vi "ADC-NEW.vi"(0 "Analog_Data(V)":dbl=0.0001 min=-15.0 max=30.0 step=0.01, 5 "Voltage_Range(V)":dbl=1.0 min=1e-06 max=30.0 step=0.01, 7 "Resolution (bits)":i32=1 min=1 max=128, 11 "Stop":bool) -> (4 "Digital_Code":i64)   [LabVIEW 2023]
doc: "This VI converts analog value into Digital value."
panel:
  # "ADC"
  # "NOTE:\n This ADC system converts -V to +V and represent the respective Digital code from -(2^(n-1)-1) to (2^(n-1)).\n\nWhere n represent the Resolution (converted for which type of system, eg 8bit, 16bit, 32bit or 64bit systems)"
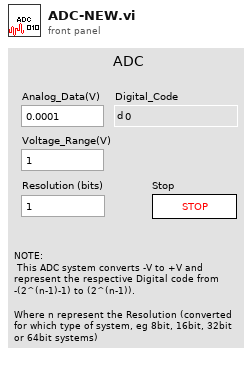
[diagram p1: front panel]
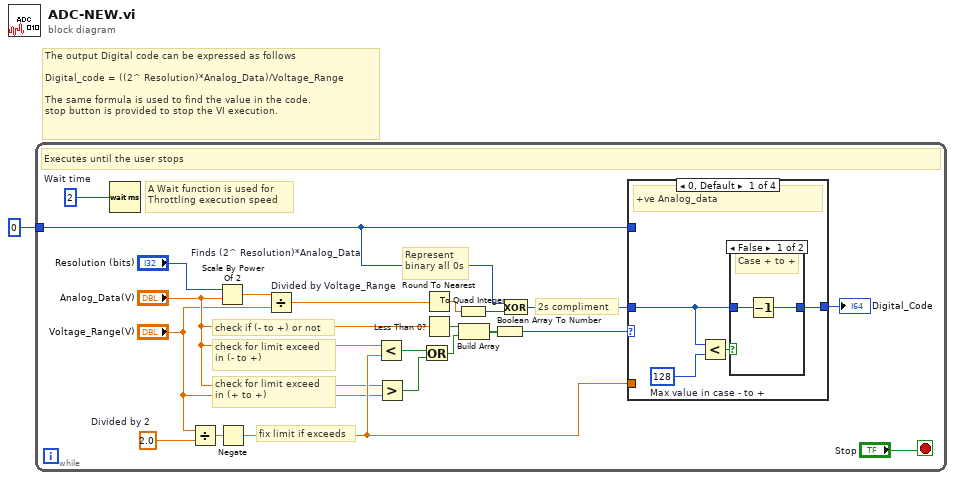
[diagram p0: block diagram]
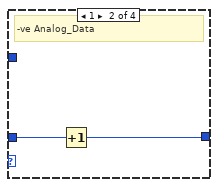
[diagram p3: hidden frame]
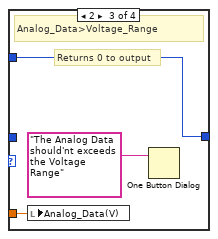
[diagram p4: hidden frame]
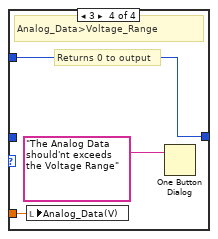
[diagram p5: hidden frame]
diagram:
  # "The output Digital code can be expressed as follows\n\nDigital_code = ((2^ Resolution)*Analog_Data)/Voltage_Range\n\nThe same formula is used to find the value in the code.\nstop button is provided to stop the VI execution."
  n1 = while {
    tunnel: i64 0 -> [w2]
    stop <- "Stop" stop-if-true
    w15 = 2.0  # Divided by 2
    w22 = u32 2  # Wait time
    # "Represent binary all 0s"
    # "check for limit exceed \nin (+ to +)"
    # "check for limit exceed \nin (- to +)"
    # "fix limit if exceeds"
    # "check if (- to +) or not"
    # "2s compliment"
    # "A Wait function is used for \nThrottling execution speed"
    # "Executes until the user stops"
    n2 = Wait (ms)(milliseconds to wait=w22) -> ()  [unwired: 1 out]
    n3 = Divide(x="Voltage_Range(V)", y=w15) -> (x/y=w10:dbl)
    n4 = Scale By Power Of 2 "Finds (2^ Resolution)*Analog_Data"(n="Resolution (bits)", x="Analog_Data(V)") -> (x*2^n=w18:dbl)
    n5 = Negate(x=w10) -> (-x=w7:dbl)
    n6 = Divide "Divided by Voltage_Range"(x=w18, y="Voltage_Range(V)") -> (x/y=w19:dbl)
    n7 = Less?(x="Analog_Data(V)", y=w7) -> (x < y?=w8:bool)
    n8 = Greater?(x="Analog_Data(V)", y="Voltage_Range(V)") -> (0:w3:bool)
    n9 = Or(x=w8, y=w3) -> (x .or. y?=w4:bool)
    n10 = Round To Nearest(number=w19) -> (nearest integer value=w20:dbl)
    n11 = Less Than 0?(x="Analog_Data(V)") -> (x < 0?=w14:bool)
    n12 = To Quad Integer(1:w20) -> (0:w9:i64)
    n13 = Build Array(w14, w4) -> (w13:bool[])
    n14 = Boolean Array To Number(Boolean array=w13) -> (number=w12:u32)
    n15 = Exclusive Or(1:w9, 2:w2) -> (0:w16:i64)
    n16 = case shown="0, Default" w12 {
      tunnel: w16 -> [w24 w31 _ _]
      tunnel: w7 -> [_ _ w33 w36]
      tunnel: [w26 w30 w32 w35] -> w11
      tunnel: w2 -> [_ _ w32 w35]
      frame 0, Default {
        w23 = i64 128  # Max value in case - to +
        # "+ve Analog_data"
        n17 = Less?(x=w24, y=w23) -> (x < y?=w25:bool)
        n18 = case shown="False" w25 {
          tunnel: [w27 w29] -> w26
          tunnel: w24 -> [w28 w29]
          frame False {
            # "Case + to +"
            n19 = Decrement(x=w28) -> (x-1=w27:i64)
          }
          frame True {
            # "Case - to+"
          }
        }
      }
      frame 1 {
        # "-ve Analog_Data"
        n20 = Increment(x=w31) -> (x+1=w30:i64)
      }
      frame 2 {
        # "Returns 0 to output"
        # "Analog_Data>Voltage_Range"
        n21 = local write "Analog_Data(V)"(w33) -> ()
        n22 = One Button Dialog(message="The Analog Data should'nt exceeds the Voltage Range") -> ()  [unwired: 1 in, 1 out]
      }
      frame 3 {
        # "Returns 0 to output"
        # "Analog_Data>Voltage_Range"
        n23 = local write "Analog_Data(V)"(w36) -> ()
        n24 = One Button Dialog(message="The Analog Data should'nt exceeds the Voltage Range") -> ()  [unwired: 1 in, 1 out]
      }
    }
    "Digital_Code" <- w11
  }
